vi "字符串转换为配置参数.vi"(1 "StringArray":string[](array[string])) -> (0 "配置参数":T1 {"积分调节时间" format="%#.1f"; "比例调节增益" format="%#.1g%%"; "速差曲线点4" format="%#.1g%%"; "速差曲线点2" format="%#.1g%%"; "速差曲线点3" format="%#.1g%%"; "速差曲线点1" format="%#.1g%%"; "速差曲线点4 反馈" format="%#.1g%%"; "速差曲线点2 反馈" format="%#.1g%%"; "速差曲线点3 反馈" format="%#.1g%%"; "速差曲线点1 反馈" format="%#.1g%%"; "最低转速" format="%#.1f"; "最高转速" format="%#.1f"; "测速盘齿数" format="%#.0f"; "DEH内置参数值" format="%.1f %"})   [LabVIEW 2013]
panel:
  # "调节参数"
  # "阀门输出"
  # "转速反馈"
  # "速差曲线点"
  # "反馈"
  # "DEH"
  # "LVDT 1"
  # "LVDT 2"
  # "DEH"
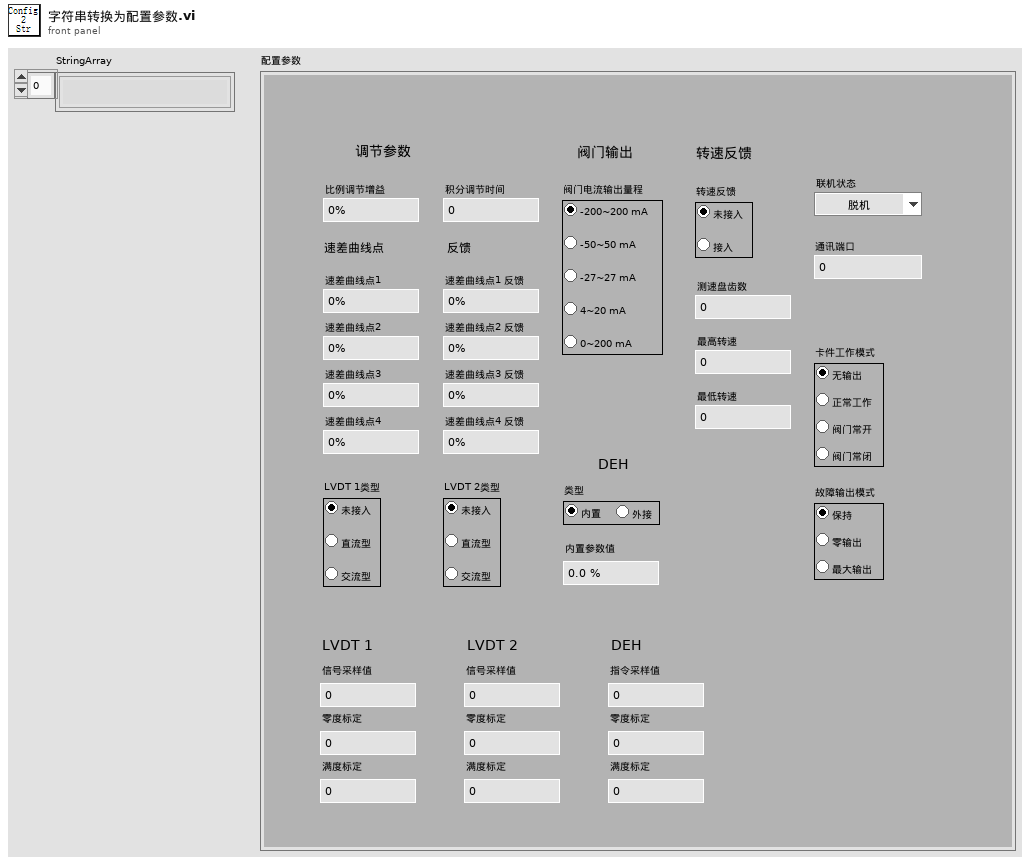
[diagram p1: front panel]
types:
  T1 = cluster{"卡件工作模式":enum32{"未接入", "直流型", "交流型", "交流型 2"}, "转速反馈":enum32{"未接入", "直流型"}, "故障输出模式":enum32{"未接入", "直流型", "交流型"}, "DEH类型":enum32{"内置", "外接"}, "LVDT 2类型":enum32{"未接入", "直流型", "交流型"}, "LVDT 1类型":enum32{"未接入", "直流型", "交流型"}, "阀门电流输出量程":enum32{"-200~200 mA", "-50~50 mA", "-27~27 mA", "4~20 mA", "0~200 mA"}, "DEH内置参数值":dbl, "测速盘齿数":dbl, "最高转速":dbl, "最低转速":dbl, "速差曲线点1 反馈":dbl, "速差曲线点3 反馈":dbl, "速差曲线点2 反馈":dbl, "速差曲线点4 反馈":dbl, "速差曲线点1":dbl, "速差曲线点3":dbl, "速差曲线点2":dbl, "速差曲线点4":dbl, "比例调节增益":dbl, "积分调节时间":dbl, "通讯端口":dbl, "联机状态":enum16{"脱机", "联机"}, "DEH零度标定":dbl, "DEH满度标定":dbl, "DEH指令采样值":dbl, "LVDT 2零度标定":dbl, "LVDT 2满度标定":dbl, "LVDT 2信号采样值":dbl, "LVDT 1零度标定":dbl, "LVDT 1满度标定":dbl, "LVDT1 信号采样值":dbl}
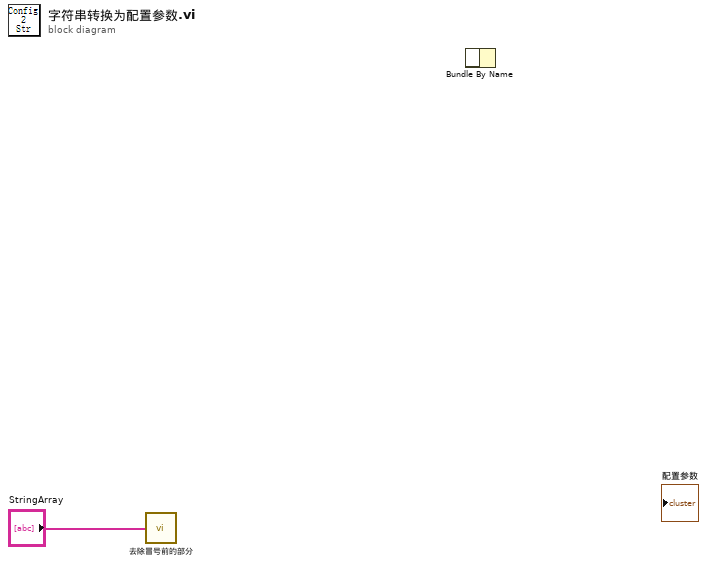
[diagram p0: block diagram]
diagram:
  n1 = call "去除冒号前的部分.vi"("返回值列表"="StringArray") -> ()  [unwired: 1 out]
  n2 = Bundle By Name() -> ()  [unwired: 2 in, 1 out]
